vi "Close KUKA youBot.vi"(8 "error in (no error)":errorcluster, 11 "KUKA youBot host in":refnum<class "NI_Robotics_KUKA youBot Host Interface.lvclass">) -> (0 "error out":errorcluster)   [LabVIEW 2017, in "NI_Robotics_KUKA youBot Host.lvlib" / "NI_Robotics_KUKA youBot Host Interface.lvclass"]
doc: "Terminates the KUKA youBot host interface."
uses:
  <vilib>/robotics/KUKA youBot/Host Interface/NI_Robotics_KUKA youBot Host Interface.lvclass
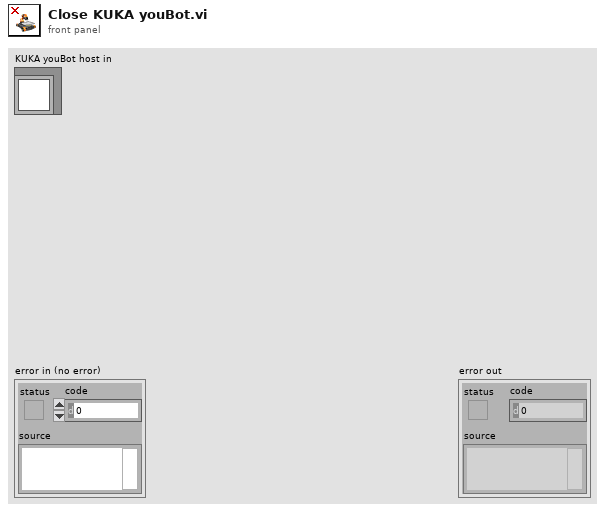
[diagram p1: front panel]
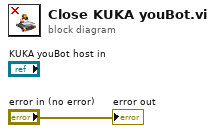
[diagram p0: block diagram]
diagram:
  "error out" <- "error in (no error)"
